vi "Test GenNet-Server API.vi"() -> ()   [LabVIEW 2014]
doc: "GenNet-Server API Tester.\n\n____\nHAMPEL SOFTWARE ENGINEERING v2.4.4 (2020-05-26 17:37)"
uses:
  UDP Broadcasting/Network Broadcast Params.ctl
  DQMH-GenNet Message Queue.lvclass
  UDP Broadcasting/Generic Broadcasts.ctl
  hse-dqmh/Dynamic Requesters/Singleton/Status Updated Argument--cluster.ctl
  hse-dqmh/Dynamic Requesters/Singleton/Error Reported Argument--cluster.ctl
  hse-dqmh/Dynamic Requesters/Singleton/Get Module Execution Status Argument--cluster.ctl
  hse-dqmh/Dynamic Requesters/Singleton/Stop Argument--cluster.ctl
  hse-dqmh/Controls/System Message Argument--cluster.ctl
  hse-dqmh/Controls/System Message Source.ctl
  GenNet-Server.lvlib
  hse-dqmh/hse-dqmh-dynamicrequesters.lvlib
  hse-dqmh/hse-dqmh.lvlib
  hse-gennet.lvlib
panel:
  in  "UDP Connection Parameters":T1
  in  "Forward Generic Broadcasts to Network":bool
  in  "Port Number":u16
  in  "Run as Singleton?":bool
  in  "Show Block Diagram":bool
  in  "Refresh Modules":bool
  out "Active Modules":string[](array[string])
  in  "Stop Module":bool
  in  "Select Module":i32(ring)=-1 caption="Select Module\nTo send Request to" items=["All"=-1]
  in  "Run New Module":bool
  in  "Hide Module Panel":bool
  in  "Show Module Panel":bool
  out "Status":string
  # "This VI tests the API for the Module."
  # "<- parameter of \"Start Module\""
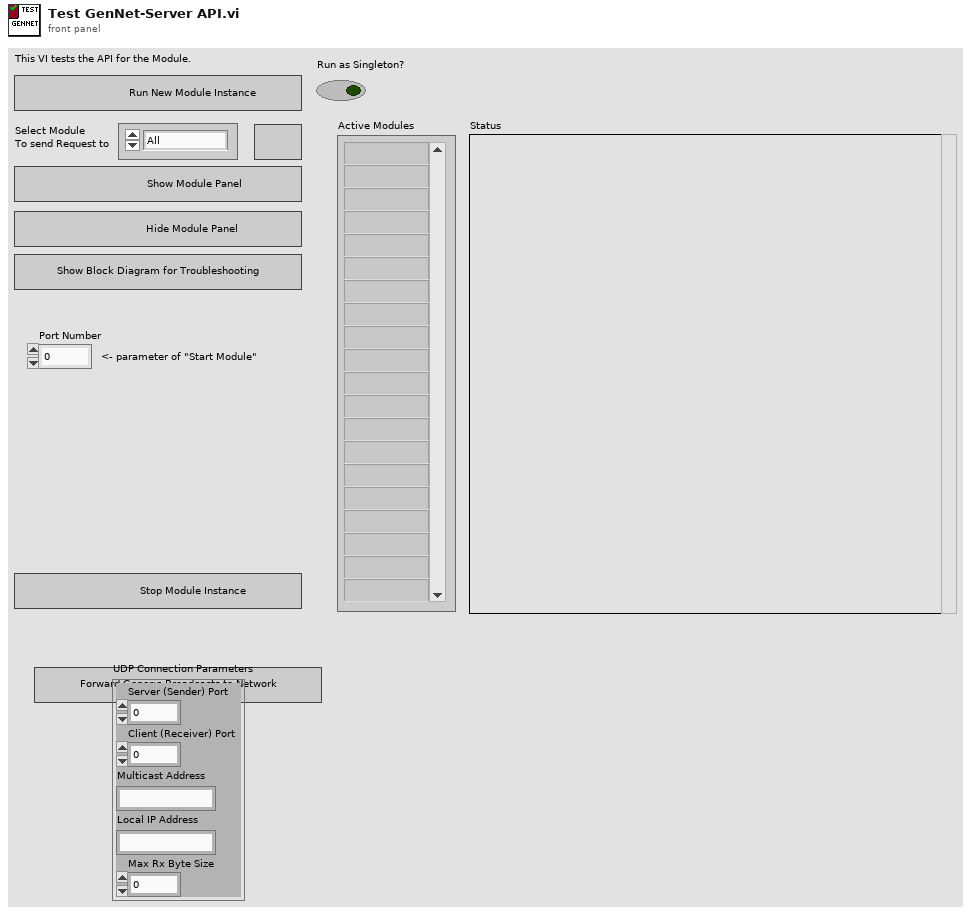
[diagram p1: front panel]
types:
  T1 = typedef "hse-gennet.lvlib/Network Broadcast Params.ctl" = cluster{"Server (Sender) Port":u16, "Client (Receiver) Port":u16, "Multicast Address":string, "Local IP Address":string, "Max Rx Byte Size":i32}
  T2 = typedef "GenNet-Server.lvlib/Broadcast Events--cluster.ctl" = cluster{"Module Did Init":refnum<user-event>, "Status Updated":refnum<user-event>, "Error Reported":refnum<user-event>, "Module Did Stop":refnum<user-event>, "Update Module Execution Status":refnum<user-event>}
  T3 = typedef "hse-gennet.lvlib/Generic Broadcasts.ctl" = cluster{"Status Updated":refnum<user-event>, "Error Reported":refnum<user-event>, "Update Module Execution Status":refnum<user-event>, "Module Did Stop":refnum<user-event>, "System Message":refnum<user-event>}
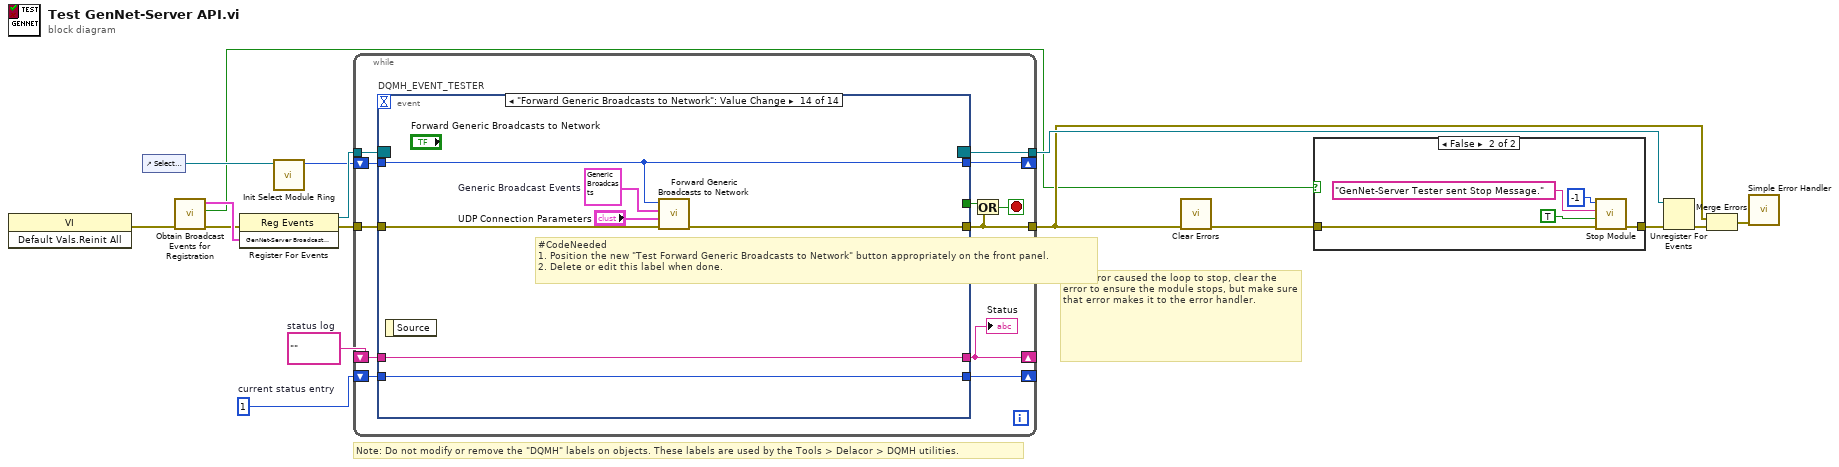
[diagram p0: block diagram]
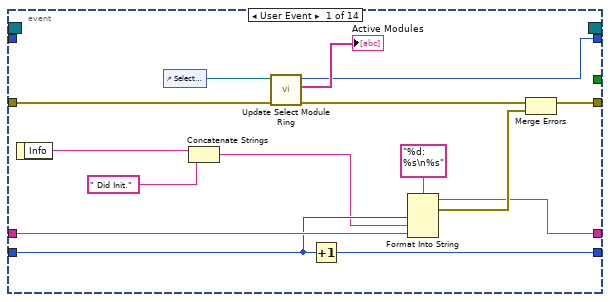
[diagram p3: hidden frame]
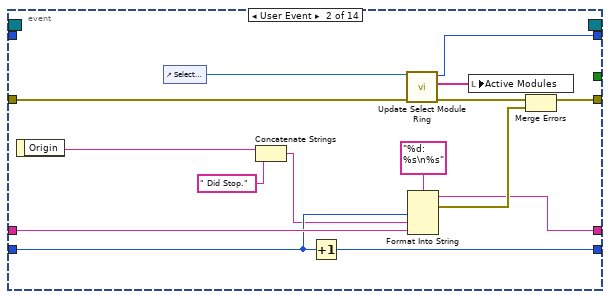
[diagram p4: hidden frame]
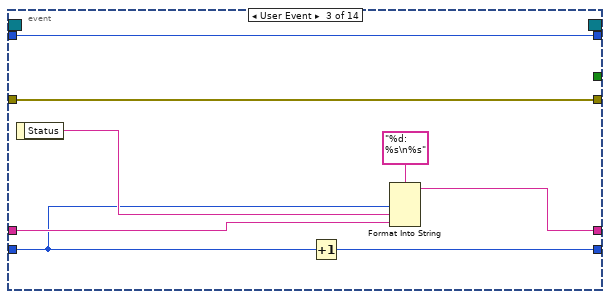
[diagram p5: hidden frame]
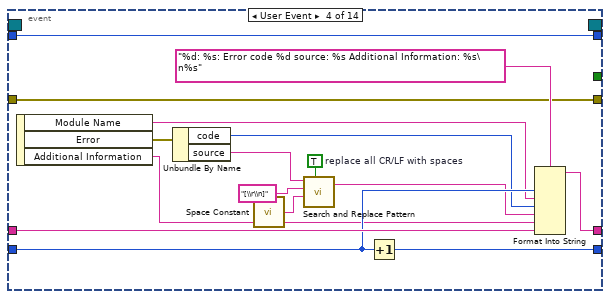
[diagram p6: hidden frame]
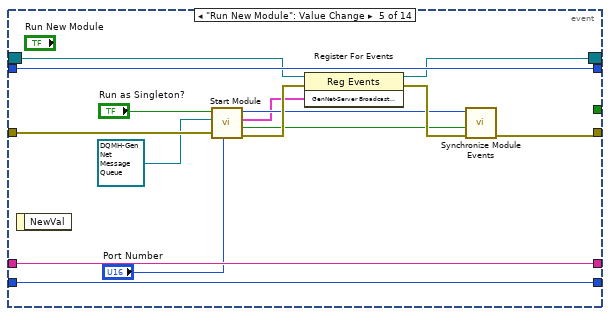
[diagram p7: hidden frame]
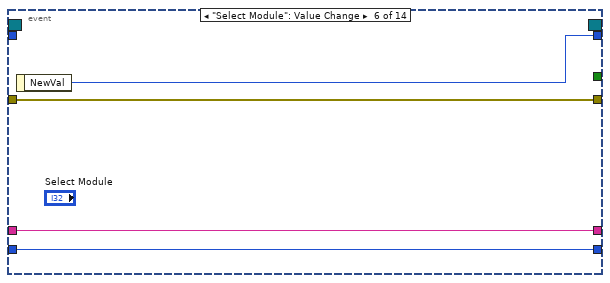
[diagram p8: hidden frame]
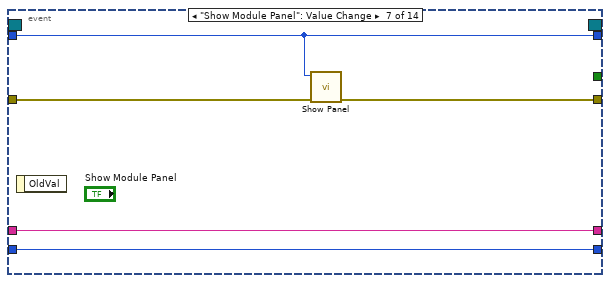
[diagram p9: hidden frame]
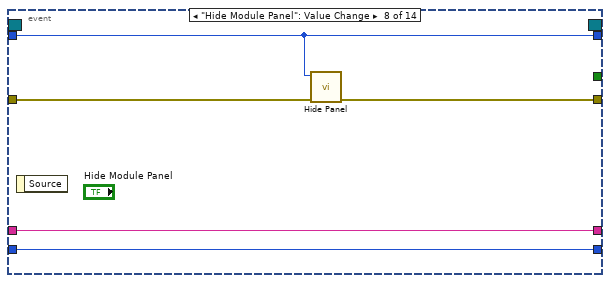
[diagram p10: hidden frame]
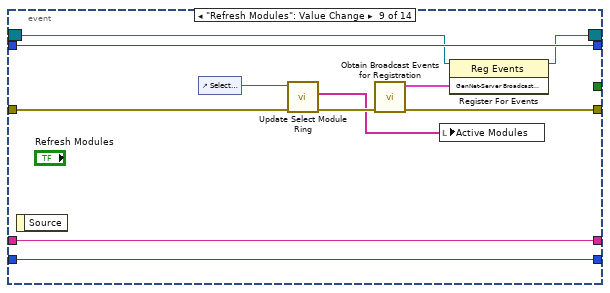
[diagram p11: hidden frame]
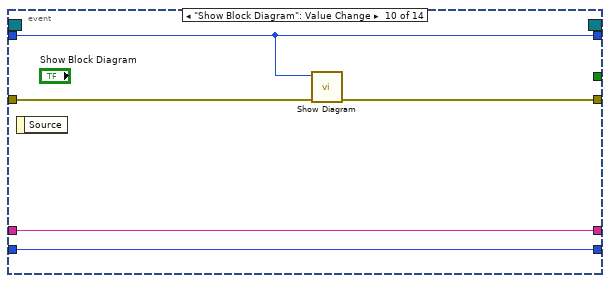
[diagram p12: hidden frame]
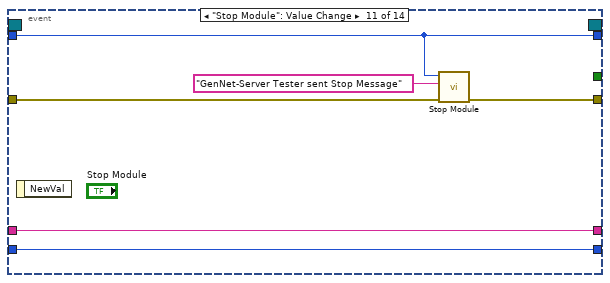
[diagram p13: hidden frame]
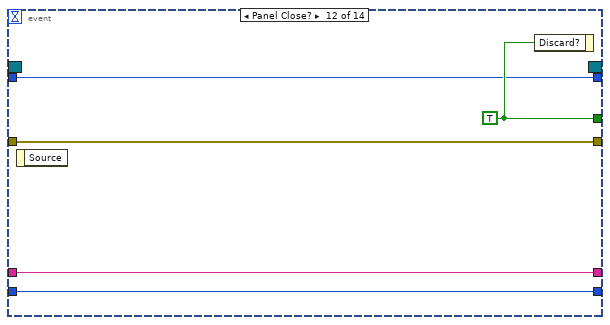
[diagram p14: hidden frame]
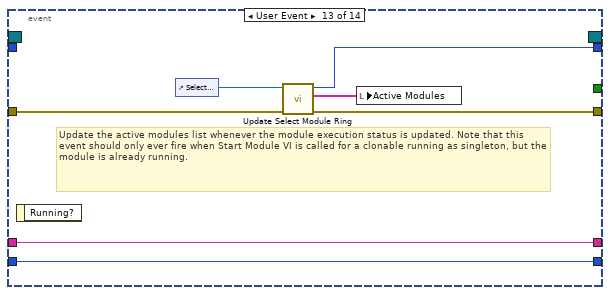
[diagram p15: hidden frame]
diagram:
  w12 = 1  # current status entry
  w13 = ""  # status log
  # "If an error caused the loop to stop, clear the error to ensure the module stops, but make sure that error makes it to the error handler."
  # "Note: Do not modify or remove the \"DQMH\" labels on objects. These labels are used by the Tools > Delacor > DQMH utilities."
  n1 = invoke class="VI" method="Default Vals.Reinit All"() -> (error out=w4:errorcluster)  [unwired: 3 in, 2 out]
  n2 = control-ref of="Select Module"() -> (w10:refnum<vi>)
  n3 = call "Obtain Broadcast Events for Registration.vi"("error in (no error)"=w4) -> ("error out"=w3:errorcluster, "Already running?"=w1:bool, "GenNet-Server Broadcast Events"=w9:T2)  [unwired: 8 in]
  n4 = register-events(error in=w3, w9) -> (reference out=w16:refnum<event-registration>, error out=w8:errorcluster)  [unwired: 1 in]
  n5 = call "Init Select Module Ring.vi"("Select Module Ring Ref"=w10) -> ("Value for All Modules"=w11:i32)  [unwired: 8 in, 2 out]
  n6 = while {
    tunnel: w16 -> [w28]
    tunnel: [w17] -> w5
    tunnel: w8 -> [w26]
    shift-right: [w22] -> _
    shift-left: w13 -> [w24]
    shift-right: [w23] -> _
    shift-left: w12 -> [w25]
    shift-right: [w19] -> _
    shift-left: w11 -> [w20]
    tunnel: [w18] -> w7
    stop <- w21 stop-if-true
    n7 = event "DQMH_EVENT_TESTER" shown="[13] \"Forward Generic Broadcasts to Network\": Value Change" {
      selector: w28 -> [_ _ _ _ w91 _ _ _ w117 _ _ _ _ _]
      dyn-events: [_ _ _ _ w90 _ _ _ w116 _ _ _ _ _] -> w18
      timeout: _ -> [_ _ _ _ _ _ _ _ _ _ _ _ _ _]
      tunnel: [_ _ _ _ _ _ _ _ _ _ _ w138 _ _] -> w27
      tunnel: [w32 w50 w66 w72 w89 w101 w105 w110 w113 w124 w129 w137 w141 w149] -> w17
      tunnel: w26 -> [w34 w52 w66 w72 w92 w101 w106 w111 w118 w127 w130 w137 w142 w152]
      tunnel: w25 -> [w40 w55 w59 w78 w94 w99 w103 w108 w121 w125 w132 w135 w144 w150]
      tunnel: w24 -> [w41 w56 w62 w80 w95 w100 w104 w109 w122 w126 w133 w136 w145 w151]
      tunnel: [w38 w53 w63 w75 w95 w100 w104 w109 w122 w126 w133 w136 w145 w151] -> w22
      tunnel: [w39 w54 w65 w81 w94 w99 w103 w108 w121 w125 w132 w135 w144 w150] -> w23
      tunnel: w20 -> [_ _ w60 w82 w93 _ w102 w107 w120 w123 w131 w134 _ w148]
      tunnel: [w29 w47 w60 w82 w93 w98 w102 w107 w120 w123 w131 w134 w140 w148] -> w19
      event User Event {
        n8 = event-data() -> ("Info"=w37:string)  [unwired: 1 in]
        n9 = control-ref of="Select Module"() -> (w31:refnum<vi>)
        n10 = Concatenate Strings(w37, " Did Init.") -> (w36:string)
        n11 = call "Update Select Module Ring.vi"("error in (no error)"=w34, "Select Module Ring Ref"=w31) -> ("error out"=w33:errorcluster, "Active Modules (Array)"=→"Active Modules":string[], "New Module Ring Value"=w29:i32)  [unwired: 7 in]
        n12 = Increment(x=w40) -> (x+1=w39:i32)
        n13 = Format Into String(format string="%d: %s\n%s", w40, w36, w41) -> (resulting string=w38:string, error out=w43:errorcluster)  [unwired: 2 in]
        n14 = Merge Errors(w33, w43) -> (w32:errorcluster)
      }
      event User Event {
        n15 = event-data() -> ("Origin"=w45:string)  [unwired: 1 in]
        n16 = control-ref of="Select Module"() -> (w49:refnum<vi>)
        n17 = Concatenate Strings(w45, " Did Stop.") -> (w44:string)
        n18 = Increment(x=w55) -> (x+1=w54:i32)
        n19 = call "Update Select Module Ring.vi"("error in (no error)"=w52, "Select Module Ring Ref"=w49) -> ("error out"=w51:errorcluster, "Active Modules (Array)"=w48:string[], "New Module Ring Value"=w47:i32)  [unwired: 7 in]
        n20 = Format Into String(format string="%d: %s\n%s", w55, w44, w56) -> (resulting string=w53:string, error out=w58:errorcluster)  [unwired: 2 in]
        n21 = local write "Active Modules"(w48) -> ()
        n22 = Merge Errors(w51, w58) -> (w50:errorcluster)
      }
      event User Event {
        n23 = event-data() -> ("Status"=w61:string)  [unwired: 1 in]
        n24 = Increment(x=w59) -> (x+1=w65:i32)
        n25 = Format Into String(format string="%d: %s\n%s", w59, w61, w62) -> (resulting string=w63:string)  [unwired: 2 in, 1 out]
      }
      event User Event {
        w76 = TRUE  # replace all CR/LF with spaces
        n26 = event-data() -> ("Module Name"=w70:string, "Error"=w69:errorcluster, "Additional Information"=w67:string)  [unwired: 1 in]
        n27 = Unbundle By Name(w69) -> ("code"=w71:i32, "source"=w73:string)
        n28 = call <vilib>:"Space Constant.vi"() -> ("String"=w77:string)
        n29 = call <vilib>:"Search and Replace Pattern.vi"("string"=w73, "regular expression (\"\")"="[\\r\\n]" ("regular expression (\"\")"), "replace string (\"\")"=w77, "replace all? (F)"=w76) -> ("result string"=w74:string)  [unwired: 1 in, 1 out]
        n30 = Increment(x=w78) -> (x+1=w81:i32)
        n31 = Format Into String(format string="%d: %s: Error code %d source: %s Additional Information: %s\n%s", w78, w70, w71, w74, w67, w80) -> (resulting string=w75:string)  [unwired: 2 in, 1 out]
      }
      event "Run New Module": Value Change {
        n32 = event-data() -> ()  [unwired: 1 in, 1 out]
        n33 = call "Start Module.vi"("Port Number"="Port Number", "error in (no error)"=w92, "Caller MsgQ"=refnum<class "DQMH-GenNet Message Queue.lvclass"> refnum, "Run as Singleton? (F)"="Run as Singleton?") -> ("error out"=w96:errorcluster, "Wait for Event Sync?"=w87:bool, "GenNet-Server Broadcast Events"=w86:T2, "Module ID"=w88:i32)  [unwired: 4 in]
        n34 = register-events(reference=w91, error in=w96, w86) -> (reference out=w90:refnum<event-registration>, error out=w97:errorcluster)
        n35 = call "Synchronize Module Events.vi"("error in (no error)"=w97, "Wait for Event Sync?"=w87, "Module ID"=w88) -> ("error out"=w89:errorcluster)  [unwired: 7 in, 1 out]
      }
      event "Select Module": Value Change {
        n36 = event-data() -> ("NewVal"=w98:i32)  [unwired: 1 in]
      }
      event "Show Module Panel": Value Change {
        n37 = event-data() -> ()  [unwired: 1 in, 1 out]
        n38 = call "Show Panel.vi"("error in (no error)"=w106, "Module ID"=w102) -> ("error out"=w105:errorcluster)  [unwired: 9 in]
      }
      event "Hide Module Panel": Value Change {
        n39 = event-data() -> ()  [unwired: 1 in, 1 out]
        n40 = call "Hide Panel.vi"("error in (no error)"=w111, "Module ID"=w107) -> ("error out"=w110:errorcluster)  [unwired: 9 in]
      }
      event "Refresh Modules": Value Change {
        n41 = event-data() -> ()  [unwired: 1 in, 1 out]
        n42 = control-ref of="Select Module"() -> (w119:refnum<vi>)
        n43 = call "Update Select Module Ring.vi"("error in (no error)"=w118, "Select Module Ring Ref"=w119) -> ("error out"=w114:errorcluster, "Active Modules (Array)"=w112:string[])  [unwired: 7 in, 1 out]
        n44 = call "Obtain Broadcast Events for Registration.vi"("error in (no error)"=w114) -> ("error out"=w113:errorcluster, "GenNet-Server Broadcast Events"=w115:T2)  [unwired: 8 in, 1 out]
        n45 = local write "Active Modules"(w112) -> ()
        n46 = register-events(reference=w117, w115) -> (reference out=w116:refnum<event-registration>)  [unwired: 1 in, 1 out]
      }
      event "Show Block Diagram": Value Change {
        n47 = event-data() -> ()  [unwired: 1 in, 1 out]
        n48 = call "Show Diagram.vi"("error in (no error)"=w127, "Module ID"=w123) -> ("error out"=w124:errorcluster)  [unwired: 9 in]
      }
      event "Stop Module": Value Change {
        n49 = event-data() -> ()  [unwired: 1 in, 1 out]
        n50 = call "Stop Module.vi"("error in (no error)"=w130, "Origin"="GenNet-Server Tester sent Stop Message", "Module ID"=w131) -> ("error out"=w129:errorcluster)  [unwired: 8 in]
      }
      event Panel Close? {
        w138 = TRUE ("Discard?")
        n51 = event-data() -> ()  [unwired: 1 in, 1 out]
        n52 = event-data("Discard?"=w138) -> ()  [unwired: 1 in, 1 out]
      }
      event User Event {
        # "Update the active modules list whenever the module execution status is updated. Note that this event should only ever fire when Start Module VI is called for a clonable running as singleton, but the module is already running."
        n53 = event-data() -> ()  [unwired: 1 in, 1 out]
        n54 = control-ref of="Select Module"() -> (w143:refnum<vi>)
        n55 = call "Update Select Module Ring.vi"("error in (no error)"=w142, "Select Module Ring Ref"=w143) -> ("error out"=w141:errorcluster, "Active Modules (Array)"=w139:string[], "New Module Ring Value"=w140:i32)  [unwired: 7 in]
        n56 = local write "Active Modules"(w139) -> ()
      }
      event "Forward Generic Broadcasts to Network": Value Change {
        w146 = T3 {"Status Updated"=refnum, "Error Reported"=refnum, "Update Module Execution Status"=refnum, "Module Did Stop"=refnum, "System Message"=refnum}  # Generic Broadcast Events
        # "#CodeNeeded\n1. Position the new \"Test Forward Generic Broadcasts to Network\" button appropriately on the front panel.\n2. Delete or edit this label when done."
        n57 = event-data() -> ()  [unwired: 1 in, 1 out]
        n58 = call "Forward Generic Broadcasts to Network.vi"("error in (no error)"=w152, "Network Broadcast Params"="UDP Connection Parameters", "Generic Broadcast Events"=w146, "Module ID"=w148) -> ("error out"=w149:errorcluster)  [unwired: 7 in]
      }
    }
    "Status" <- w22
    n59 = Or(x=w27, y=w17) -> (x .or. y?=w21:bool)
  }
  n60 = call <vilib>:"Clear Errors.vi"("error in (no error)"=w5) -> ("error out"=w6:errorcluster)  [unwired: 5 in, 1 out]
  n61 = case shown="False" w1 {
    tunnel: [w153 w158] -> w14
    tunnel: w6 -> [w153 w155]
    frame True {
    }
    frame False {
      n62 = call "Stop Module.vi"("error in (no error)"=w155, "Wait for Module to stop? (F)"=TRUE ("Wait for Module to stop?"), "Origin"="GenNet-Server Tester sent Stop Message.", "Module ID"=-1) -> ("error out"=w158:errorcluster)  [unwired: 7 in]
    }
  }
  n63 = Unregister For Events(event registration refnum=w7, error in=w14) -> (error out=w15:errorcluster)
  n64 = Merge Errors(w5, w15) -> (w2:errorcluster)
  n65 = call <vilib>:"Simple Error Handler.vi"("error in (no error)"=w2) -> ()  [unwired: 4 in, 5 out]
